vi "Save-Recall Random Memory.vi"(8 "error in (no error)":errorcluster, 10 "Operation (0: Save)":u16(ring) items=["Save", "Recall"], 11 "VISA resource name":refnum<visa-resource-name>) -> (0 "error out":errorcluster, 3 "VISA resource name out":refnum<visa-resource-name>)   [LabVIEW 2017, in "ADCMT 6240.lvlib"]
doc: "This VI saves or recalls the random sweep memory data.\nAll the memories are saved or recalled regardless of a function."
uses:
  ADCMT 6240.lvlib
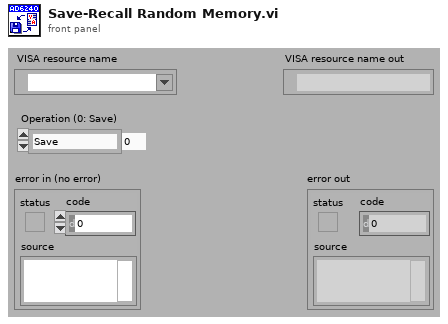
[diagram p1: front panel]
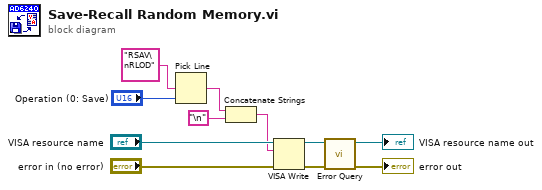
[diagram p0: block diagram]
diagram:
  n1 = Pick Line(multi-line string="RSAV\nRLOD", line index="Operation (0: Save)") -> (output string=w2:string)  [unwired: 1 in]
  n2 = Concatenate Strings(w2, "\n") -> (w1:string)
  n3 = VISA Write(VISA resource name="VISA resource name", write buffer=w1, error in (no error)="error in (no error)") -> (VISA resource name out=w7:refnum<visa-resource-name>, error out=w6:errorcluster)  [unwired: 1 out]
  n4 = call "Error Query.vi"("error in (no error)"=w6, "VISA resource name"=w7) -> ("error out"=→"error out":errorcluster, "VISA resource name out"=→"VISA resource name out":refnum<visa-resource-name>)  [unwired: 6 in, 2 out]
